vi "sTRING2.vi"(6 "angulo":dbl, 7 "Orden":T1(array[ring])=[enum."espejos", enum."voltaje", enum."polarizador", enum."potenciometro "], 8 "Valor del voltaje":dbl, 9 "cadena entrada":string, 10 "corriente":dbl) -> (2 "String":string)   [LabVIEW 2016]
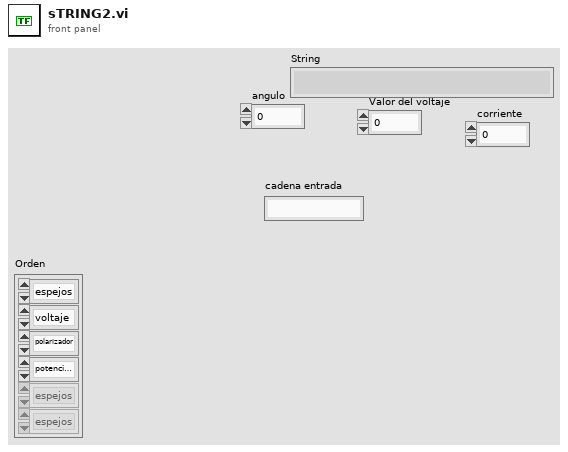
[diagram p1: front panel]
types:
  T1 = enum16{"espejos", "polarizador", "voltaje", "potenciometro ", "CCD", "lockin", "laser", "ninguno"}[]
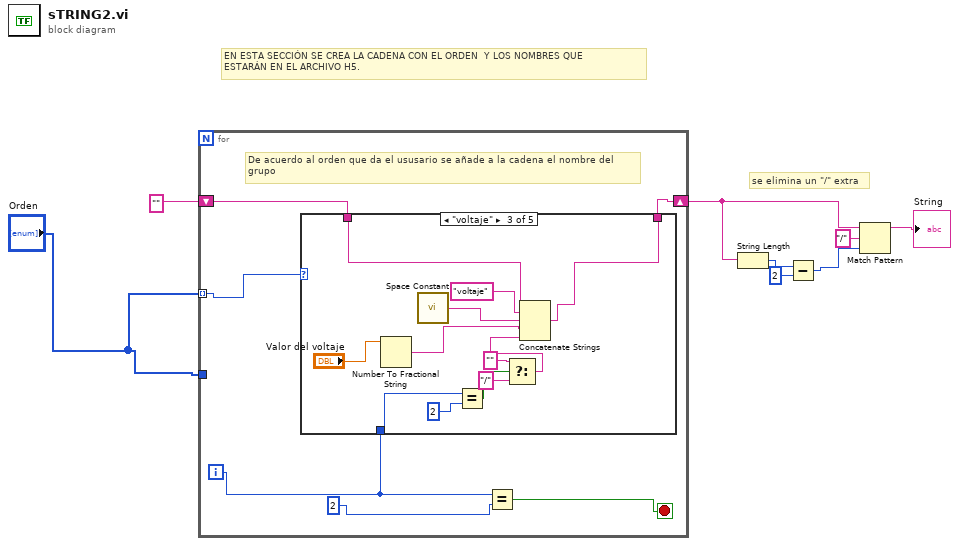
[diagram p0: block diagram]
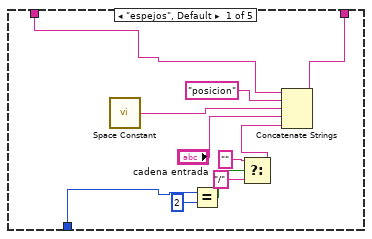
[diagram p2: hidden frame]
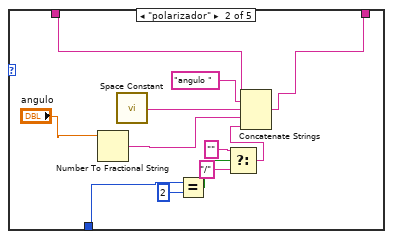
[diagram p3: hidden frame]
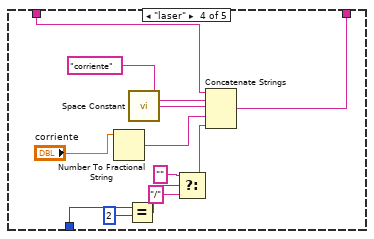
[diagram p4: hidden frame]
diagram:
  # "se elimina un \"/\" extra"
  # "EN ESTA SECCIÓN SE CREA LA CADENA CON EL ORDEN  Y LOS NOMBRES QUE \nESTARÁN EN EL ARCHIVO H5."
  n1 = for {
    tunnel: "Orden" -> [w13] mode=indexing
    shift-right: [w11] -> w6
    shift-left: "" -> [w12]
    tunnel: "Orden" -> [_]
    i -> [w10]
    stop <- w14 stop-if-true
    # "De acuerdo al orden que da el ususario se añade a la cadena el nombre del\ngrupo"
    n2 = case shown="\"voltaje\"" w13 {
      tunnel: w12 -> [w25 w36 w49 w61 w62]
      tunnel: [w24 w35 w48 w53 w62] -> w11
      tunnel: w10 -> [w23 w37 w47 w55 _]
      frame "espejos", Default {
        n3 = call <vilib>:"Space Constant.vi"() -> ("String"=w15:string)
        n4 = Equal?(x=w23, y=2) -> (x = y?=w20:bool)
        n5 = Select(t="", s=w20, f="/") -> (s? t:f=w17:string)
        n6 = Concatenate Strings(w25, "posicion", w15, "cadena entrada", w17) -> (w24:string)
      }
      frame "polarizador" {
        n7 = Number To Fractional String(number="angulo") -> (F-format string=w27:string)  [unwired: 3 in]
        n8 = call <vilib>:"Space Constant.vi"() -> ("String"=w26:string)
        n9 = Equal?(x=w37, y=2) -> (x = y?=w31:bool)
        n10 = Select(t="", s=w31, f="/") -> (s? t:f=w28:string)
        n11 = Concatenate Strings(w36, "angulo ", w26, w27, w28) -> (w35:string)
      }
      frame "voltaje" {
        n12 = Number To Fractional String(number="Valor del voltaje") -> (F-format string=w39:string)  [unwired: 3 in]
        n13 = call <vilib>:"Space Constant.vi"() -> ("String"=w38:string)
        n14 = Equal?(x=w47, y=2) -> (x = y?=w43:bool)
        n15 = Select(t="", s=w43, f="/") -> (s? t:f=w40:string)
        n16 = Concatenate Strings(w49, "voltaje", w38, w39, w40) -> (w48:string)
      }
      frame "laser" {
        n17 = Number To Fractional String(number="corriente") -> (F-format string=w51:string)  [unwired: 3 in]
        n18 = Equal?(x=w55, y=2) -> (x = y?=w58:bool)
        n19 = call <vilib>:"Space Constant.vi"() -> ("String"=w50:string)
        n20 = Select(t="", s=w58, f="/") -> (s? t:f=w52:string)
        n21 = Concatenate Strings(w61, "corriente" ("string"), w50, w51, w52) -> (w53:string)
      }
      frame "ninguno" {
      }
    }
    n22 = Equal?(x=w10, y=2 ("t")) -> (x = y?=w14:bool)
  }
  n23 = String Length(string=w6) -> (length=w5:i32)
  n24 = Subtract(x=w5, y=2) -> (x-y=w3:i32)
  n25 = Match Pattern(string=w6, regular expression="/", offset (0)=w3) -> (before substring=→"String":string)  [unwired: 3 out]
